vi "simple_cache_analog.vi"(1 "refresh":bool, 2 "new_val":fxp<+/-,24,5>) -> (0 "$_val":fxp<+/-,24,5>)   [LabVIEW 2018]
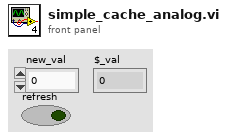
[diagram p1: front panel]
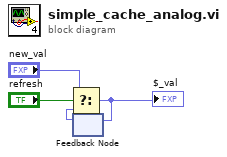
[diagram p0: block diagram]
diagram:
  n1 = feedback #1() -> (w1:fxp<+/-,24,5>)  [unwired: 1 in]
  n2 = Select(t="new_val", s="refresh", f=w1) -> (s? t:f=w2:fxp<+/-,24,5>)
  "$_val" <- w2
  n3 = feedback-in #1(w2) -> ()
